vi "Init.vi"(10 "Event":refnum<class "Event.lvclass">) -> (3 "Last Ack Event Msg Strategy out":refnum<class "Last Ack Event Msg Strategy.lvclass">)   [LabVIEW 2021, in "jettl.lvlib" / "jettl Msg Last Ack Event.lvlib" / "Last Ack Event Msg Strategy.lvclass"]
uses:
  Last Ack Event Msg Strategy.lvclass
  Event/Event.lvclass
  Last Ack Event Msg Strategy.lvclass/Last Ack Event Msg Strategy.ctl
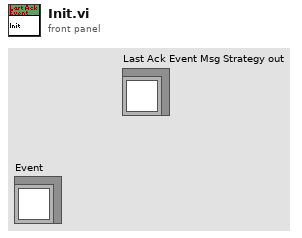
[diagram p1: front panel]
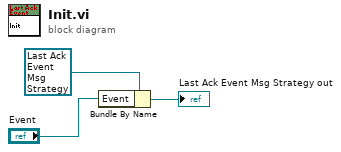
[diagram p0: block diagram]
diagram:
  n1 = Bundle By Name(cluster=refnum<class "Last Ack Event Msg Strategy.lvclass"> refnum ("Event Last Ack Msg out"), "Event"="Event") -> (→"Last Ack Event Msg Strategy out":refnum<class "Last Ack Event Msg Strategy.lvclass">)
